vi "Facade.vi"(0 "Data In":T4, 2 "Display State In":T2, 3 "Container State":T3) -> (6 "Data Out":T4, 7 "Display State Out":T2, 8 "Action":T1)   [LabVIEW 2015, in "ToneCloud.xctl"]
uses:
  ToneCloud.xctl
  Data.vi
  Classes/Waveforms/Tone Cloud/Tone Cloud.lvclass
  <vilib>/_xctls/Container State.ctl
  State.vi
  <vilib>/_xctls/Action.ctl
  Classes/Waveforms/Tone Cloud/Tone Cloud.lvclass/Tone Cloud.ctl
  Classes/Waveforms/Tone Cloud/Read Serialized.vi
  Classes/Waveforms/Tone Cloud/Write Serialized.vi
  <vilib>/_xctls/XControlSupport.lvlib
panel:
  in  "Plot mask":bool
  in  "Tokens":i32 min=0
  in  "Seed":i32
  in  "Rate (Hz)":dbl
  in  "Duration (ms)":dbl
  in  "Ramp (ms)":dbl
  in  "Density":string
  in  "Level mode":enum16{"per component", "total rms"}(ring)
  in  "Level (dB)":string
  in  "#/oct":dbl=1.0 min=1.0
  in  "Spacing":enum16{"Linear", "Log"}(ring)
  in  "Fmax (Hz)":dbl
  in  "Fmin (Hz)":dbl
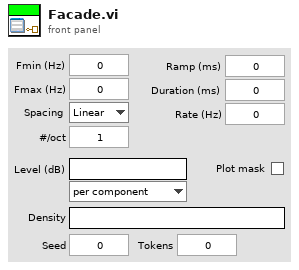
[diagram p1: front panel]
types:
  T1 = typedef "XControlSupport.lvlib/Action.ctl" = cluster{"Data Changed?":bool, "State Changed?":bool, "Action Name":string}
  T2 = typedef "ToneCloud.xctl/State.vi" = cluster{"Numeric":dbl}
  T3 = typedef "XControlSupport.lvlib/Container State.ctl" = cluster{"Indicator?":bool, "Run Mode?":bool, " Refnum":refnum<vi>}
  T4 = typedef "ToneCloud.xctl/Data.vi" = refnum<class "Tone Cloud.lvclass">
  T5 = typedef "Tone Cloud.lvclass/Serialized.ctl" = cluster{"Fmin (Hz)":dbl, "Fmax (Hz)":dbl, "Spacing":T6, "Components/oct":dbl, "Level (dB)":string, "Level mode":T7, "Density":string, "Pip ramp (ms)":dbl, "Pip duration (ms)":dbl, "Pip rate (Hz)":dbl, "Seed":i32, "Tokens":i32, "Plot mask":bool}
  T6 = typedef "Tone Cloud.lvclass/Spacing.ctl" = enum16{"Linear", "Log"}
  T7 = typedef "Tone Cloud.lvclass/Level Mode.ctl" = enum16{"per component", "total rms"}
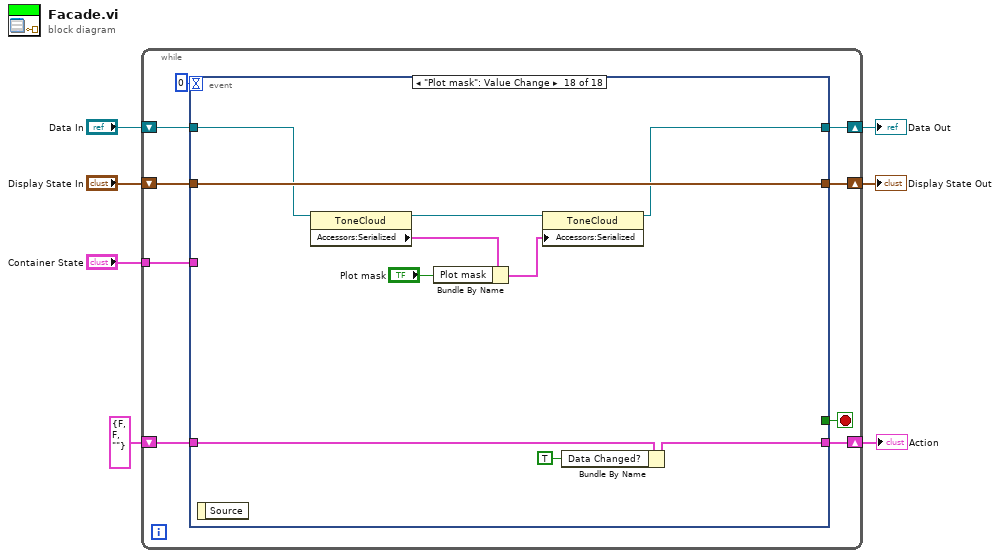
[diagram p0: block diagram]
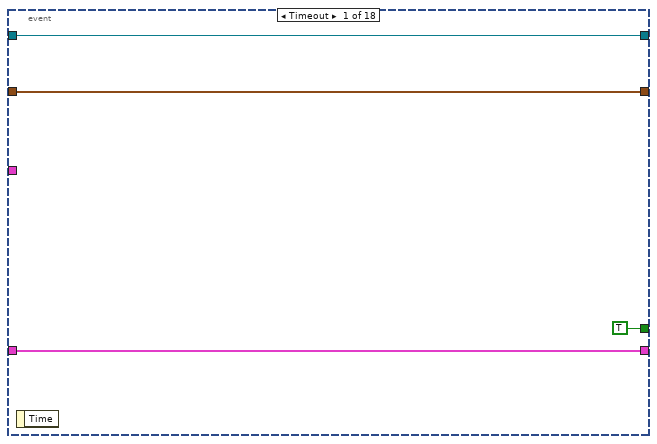
[diagram p2: hidden frame]
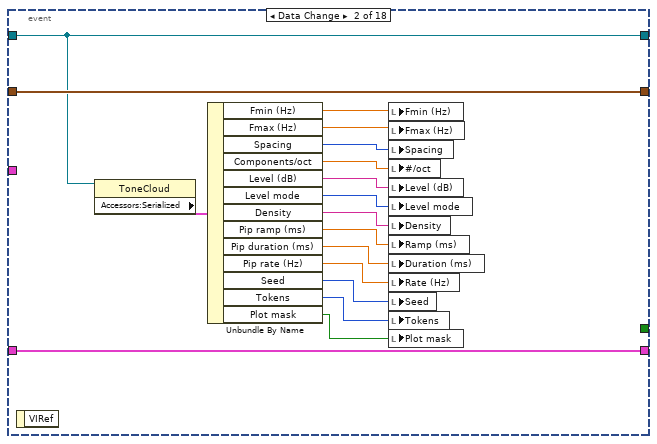
[diagram p3: hidden frame]
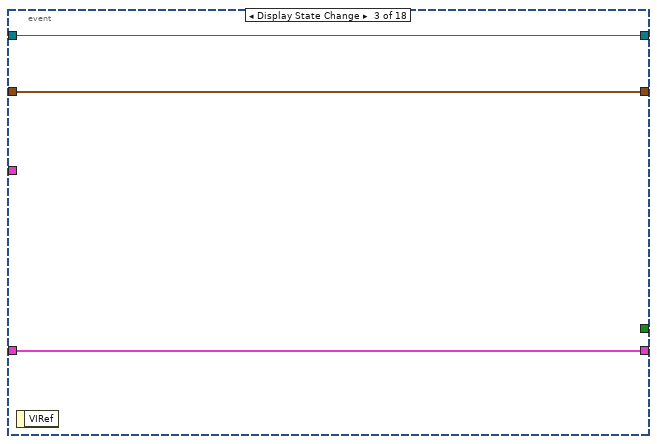
[diagram p4: hidden frame]
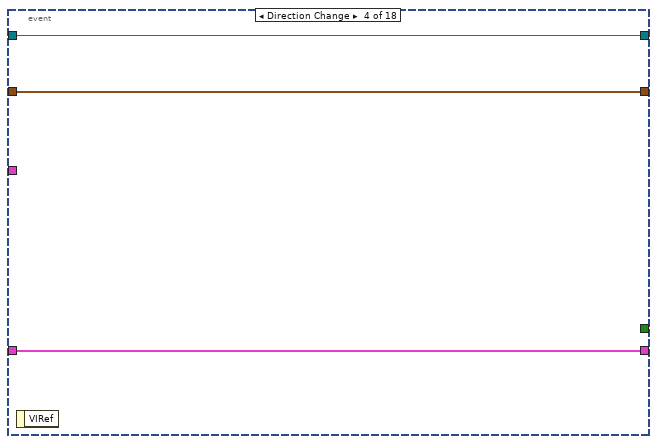
[diagram p5: hidden frame]
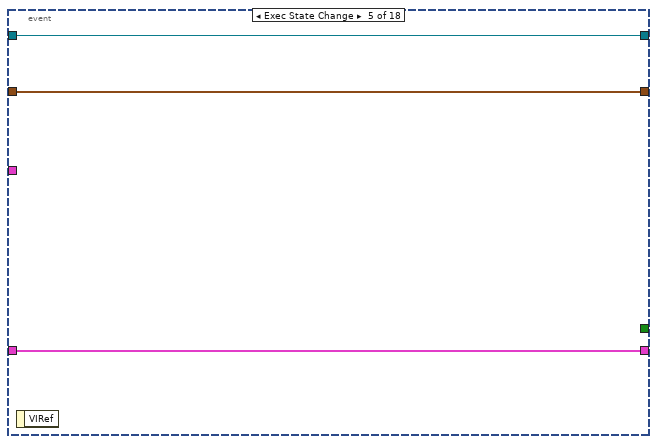
[diagram p6: hidden frame]
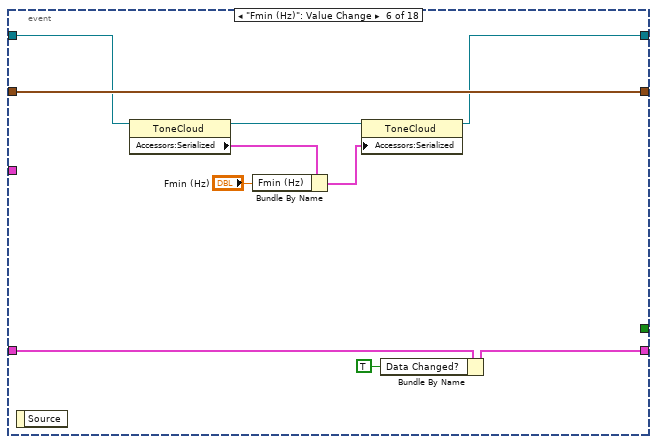
[diagram p7: hidden frame]
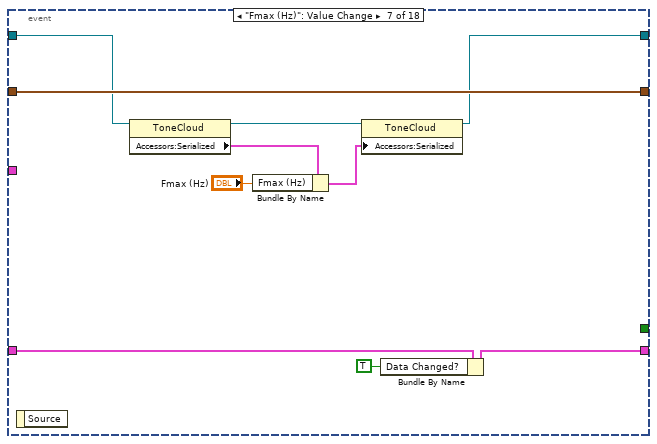
[diagram p8: hidden frame]
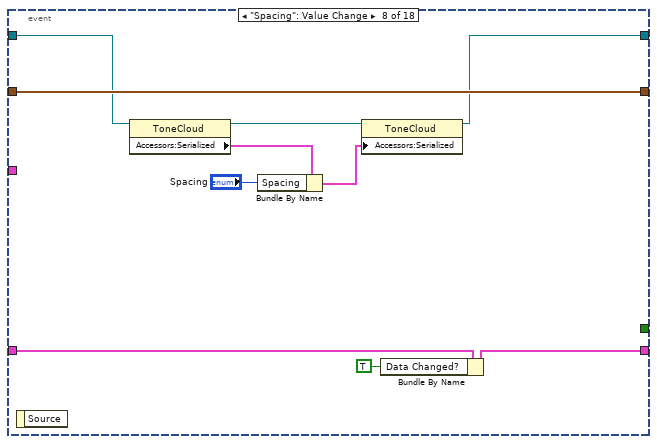
[diagram p9: hidden frame]
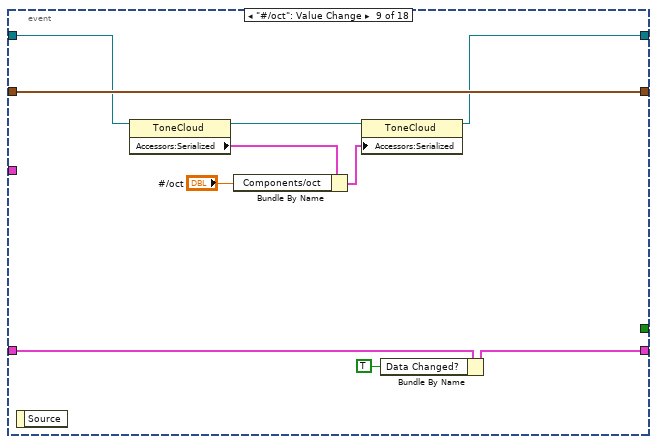
[diagram p10: hidden frame]
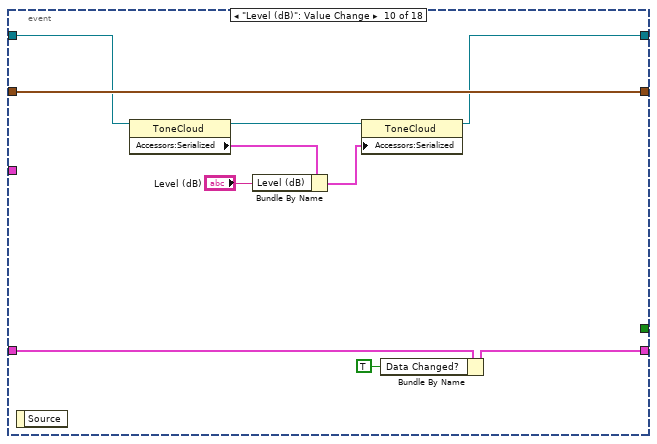
[diagram p11: hidden frame]
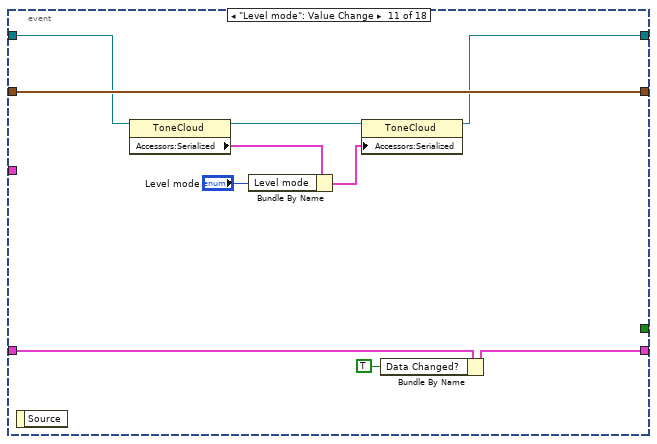
[diagram p12: hidden frame]
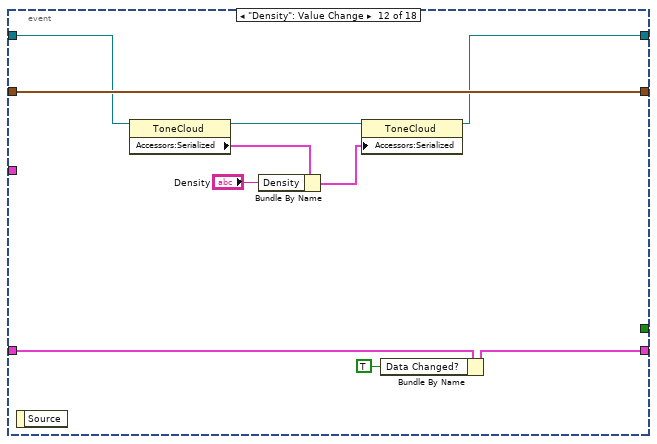
[diagram p13: hidden frame]
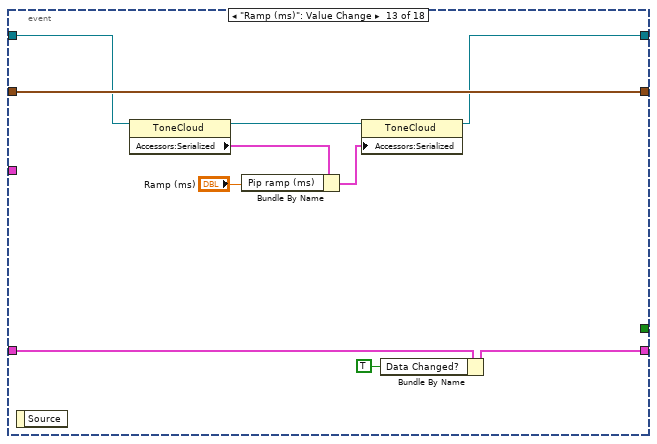
[diagram p14: hidden frame]
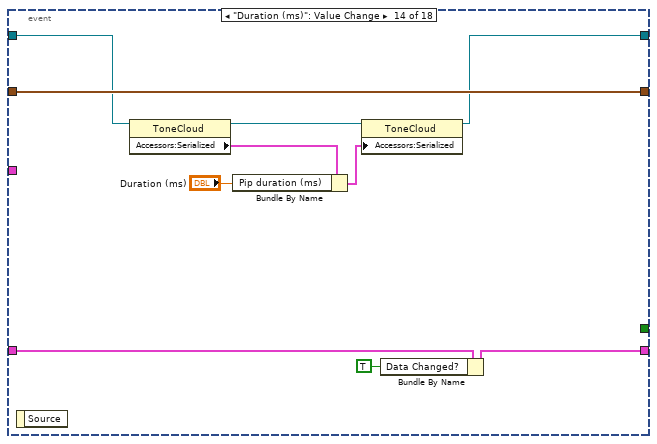
[diagram p15: hidden frame]
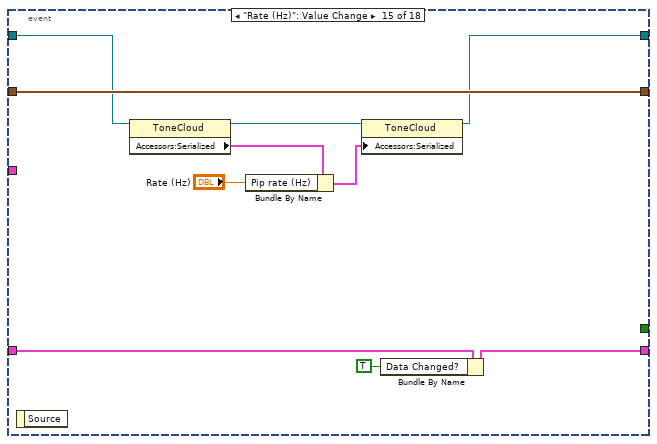
[diagram p16: hidden frame]
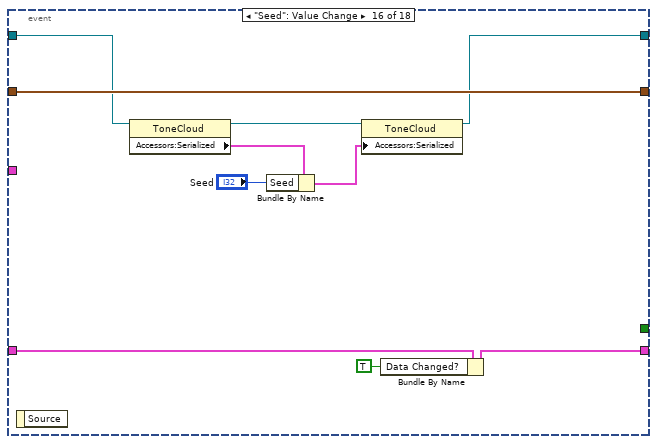
[diagram p17: hidden frame]
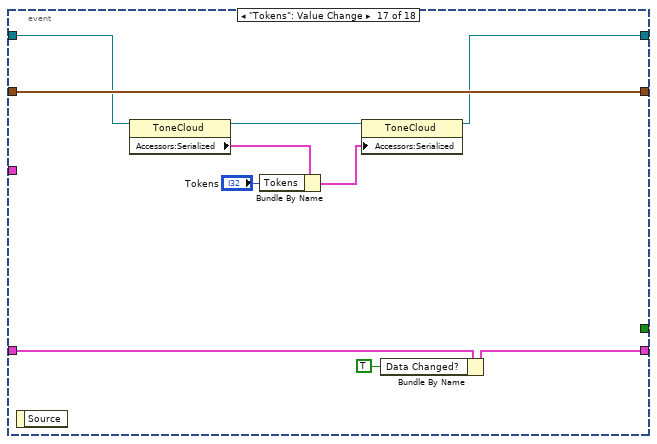
[diagram p18: hidden frame]
diagram:
  n1 = while {
    shift-right: [w15] -> w4
    shift-left: "Display State In" -> [w16]
    tunnel: "Container State" -> [w12]
    shift-right: [w10] -> w7
    shift-left: "Data In" -> [w11]
    shift-right: [w8] -> w2
    shift-left: T1 {"Data Changed?"=FALSE, "State Changed?"=FALSE, "Action Name"=""} ("Action") -> [w9]
    stop <- w14 stop-if-true
    n2 = event shown="[17] \"Plot mask\": Value Change" {
      selector: _ -> [_ _ _ _ _ _ _ _ _ _ _ _ _ _ _ _ _ _]
      dyn-events: _ -> [_ _ _ _ _ _ _ _ _ _ _ _ _ _ _ _ _ _]
      timeout: 0 -> [_ _ _ _ _ _ _ _ _ _ _ _ _ _ _ _ _ _]
      tunnel: w16 -> [w18 w37 w40 w43 w46 w56 w66 w76 w86 w96 w106 w116 w126 w136 w146 w156 w166 w176]
      tunnel: [w18 w37 w40 w43 w46 w56 w66 w76 w86 w96 w106 w116 w126 w136 w146 w156 w166 w176] -> w15
      tunnel: [TRUE _ _ _ _ _ _ _ _ _ _ _ _ _ _ _ _ _] -> w14
      tunnel: w12 -> [_ _ _ _ _ _ _ _ _ _ _ _ _ _ _ _ _ _]
      tunnel: w11 -> [w17 w35 w39 w42 w45 w49 w59 w69 w79 w89 w99 w109 w119 w129 w139 w149 w159 w169]
      tunnel: [w17 w35 w39 w42 w45 w48 w58 w68 w78 w88 w98 w108 w118 w128 w138 w148 w158 w168] -> w10
      tunnel: [w19 w36 w38 w41 w44 w54 w64 w74 w84 w94 w104 w114 w124 w134 w144 w154 w164 w174] -> w8
      tunnel: w9 -> [w19 w36 w38 w41 w44 w55 w65 w75 w85 w95 w105 w115 w125 w135 w145 w155 w165 w175]
      event Timeout {
        n3 = event-data() -> ()  [unwired: 1 in, 1 out]
      }
      event Data Change {
        n4 = event-data() -> ()  [unwired: 1 in, 1 out]
        n5 = property class="ToneCloud"(reference=w35) -> ("Accessors:Serialized"=w34:T5)  [unwired: 1 in, 2 out]
        n6 = Unbundle By Name(w34) -> ("Fmin (Hz)"=w33:dbl, "Fmax (Hz)"=w32:dbl, "Spacing"=w31:T6, "Components/oct"=w30:dbl, "Level (dB)"=w29:string, "Level mode"=w28:T7, "Density"=w27:string, "Pip ramp (ms)"=w26:dbl, "Pip duration (ms)"=w25:dbl, "Pip rate (Hz)"=w24:dbl, "Seed"=w23:i32, "Tokens"=w22:i32, "Plot mask"=w21:bool)
        n7 = local write "Fmin (Hz)"(w33) -> ()
        n8 = local write "Fmax (Hz)"(w32) -> ()
        n9 = local write "Spacing"(w31) -> ()
        n10 = local write "#/oct"(w30) -> ()
        n11 = local write "Level (dB)"(w29) -> ()
        n12 = local write "Level mode"(w28) -> ()
        n13 = local write "Density"(w27) -> ()
        n14 = local write "Ramp (ms)"(w26) -> ()
        n15 = local write "Duration (ms)"(w25) -> ()
        n16 = local write "Rate (Hz)"(w24) -> ()
        n17 = local write "Seed"(w23) -> ()
        n18 = local write "Tokens"(w22) -> ()
        n19 = local write "Plot mask"(w21) -> ()
      }
      event Display State Change {
        n20 = event-data() -> ()  [unwired: 1 in, 1 out]
      }
      event Direction Change {
        n21 = event-data() -> ()  [unwired: 1 in, 1 out]
      }
      event Exec State Change {
        n22 = event-data() -> ()  [unwired: 1 in, 1 out]
      }
      event "Fmin (Hz)": Value Change {
        n23 = event-data() -> ()  [unwired: 1 in, 1 out]
        n24 = property class="ToneCloud"(reference=w49) -> (reference out=w51:T4, "Accessors:Serialized"=w52:T5)  [unwired: 1 in, 1 out]
        n25 = Bundle By Name(cluster=w52, "Fmin (Hz)"="Fmin (Hz)") -> (w50:T5)
        n26 = property class="ToneCloud"(reference=w51, "Accessors:Serialized"=w50) -> (reference out=w48:T4)  [unwired: 1 in, 1 out]
        n27 = Bundle By Name(cluster=w55, "Data Changed?"=TRUE) -> (w54:T1)
      }
      event "Fmax (Hz)": Value Change {
        n28 = event-data() -> ()  [unwired: 1 in, 1 out]
        n29 = property class="ToneCloud"(reference=w59) -> (reference out=w61:T4, "Accessors:Serialized"=w62:T5)  [unwired: 1 in, 1 out]
        n30 = Bundle By Name(cluster=w62, "Fmax (Hz)"="Fmax (Hz)") -> (w60:T5)
        n31 = property class="ToneCloud"(reference=w61, "Accessors:Serialized"=w60) -> (reference out=w58:T4)  [unwired: 1 in, 1 out]
        n32 = Bundle By Name(cluster=w65, "Data Changed?"=TRUE) -> (w64:T1)
      }
      event "Spacing": Value Change {
        n33 = event-data() -> ()  [unwired: 1 in, 1 out]
        n34 = property class="ToneCloud"(reference=w69) -> (reference out=w71:T4, "Accessors:Serialized"=w72:T5)  [unwired: 1 in, 1 out]
        n35 = Bundle By Name(cluster=w72, "Spacing"="Spacing") -> (w70:T5)
        n36 = property class="ToneCloud"(reference=w71, "Accessors:Serialized"=w70) -> (reference out=w68:T4)  [unwired: 1 in, 1 out]
        n37 = Bundle By Name(cluster=w75, "Data Changed?"=TRUE) -> (w74:T1)
      }
      event "#/oct": Value Change {
        n38 = event-data() -> ()  [unwired: 1 in, 1 out]
        n39 = property class="ToneCloud"(reference=w79) -> (reference out=w81:T4, "Accessors:Serialized"=w82:T5)  [unwired: 1 in, 1 out]
        n40 = Bundle By Name(cluster=w82, "Components/oct"="#/oct") -> (w80:T5)
        n41 = property class="ToneCloud"(reference=w81, "Accessors:Serialized"=w80) -> (reference out=w78:T4)  [unwired: 1 in, 1 out]
        n42 = Bundle By Name(cluster=w85, "Data Changed?"=TRUE) -> (w84:T1)
      }
      event "Level (dB)": Value Change {
        n43 = event-data() -> ()  [unwired: 1 in, 1 out]
        n44 = property class="ToneCloud"(reference=w89) -> (reference out=w91:T4, "Accessors:Serialized"=w92:T5)  [unwired: 1 in, 1 out]
        n45 = Bundle By Name(cluster=w92, "Level (dB)"="Level (dB)") -> (w90:T5)
        n46 = property class="ToneCloud"(reference=w91, "Accessors:Serialized"=w90) -> (reference out=w88:T4)  [unwired: 1 in, 1 out]
        n47 = Bundle By Name(cluster=w95, "Data Changed?"=TRUE) -> (w94:T1)
      }
      event "Level mode": Value Change {
        n48 = event-data() -> ()  [unwired: 1 in, 1 out]
        n49 = property class="ToneCloud"(reference=w99) -> (reference out=w101:T4, "Accessors:Serialized"=w102:T5)  [unwired: 1 in, 1 out]
        n50 = Bundle By Name(cluster=w102, "Level mode"="Level mode") -> (w100:T5)
        n51 = property class="ToneCloud"(reference=w101, "Accessors:Serialized"=w100) -> (reference out=w98:T4)  [unwired: 1 in, 1 out]
        n52 = Bundle By Name(cluster=w105, "Data Changed?"=TRUE) -> (w104:T1)
      }
      event "Density": Value Change {
        n53 = event-data() -> ()  [unwired: 1 in, 1 out]
        n54 = property class="ToneCloud"(reference=w109) -> (reference out=w111:T4, "Accessors:Serialized"=w112:T5)  [unwired: 1 in, 1 out]
        n55 = Bundle By Name(cluster=w112, "Density"="Density") -> (w110:T5)
        n56 = property class="ToneCloud"(reference=w111, "Accessors:Serialized"=w110) -> (reference out=w108:T4)  [unwired: 1 in, 1 out]
        n57 = Bundle By Name(cluster=w115, "Data Changed?"=TRUE) -> (w114:T1)
      }
      event "Ramp (ms)": Value Change {
        n58 = event-data() -> ()  [unwired: 1 in, 1 out]
        n59 = property class="ToneCloud"(reference=w119) -> (reference out=w121:T4, "Accessors:Serialized"=w122:T5)  [unwired: 1 in, 1 out]
        n60 = Bundle By Name(cluster=w122, "Pip ramp (ms)"="Ramp (ms)") -> (w120:T5)
        n61 = property class="ToneCloud"(reference=w121, "Accessors:Serialized"=w120) -> (reference out=w118:T4)  [unwired: 1 in, 1 out]
        n62 = Bundle By Name(cluster=w125, "Data Changed?"=TRUE) -> (w124:T1)
      }
      event "Duration (ms)": Value Change {
        n63 = event-data() -> ()  [unwired: 1 in, 1 out]
        n64 = property class="ToneCloud"(reference=w129) -> (reference out=w131:T4, "Accessors:Serialized"=w132:T5)  [unwired: 1 in, 1 out]
        n65 = Bundle By Name(cluster=w132, "Pip duration (ms)"="Duration (ms)") -> (w130:T5)
        n66 = property class="ToneCloud"(reference=w131, "Accessors:Serialized"=w130) -> (reference out=w128:T4)  [unwired: 1 in, 1 out]
        n67 = Bundle By Name(cluster=w135, "Data Changed?"=TRUE) -> (w134:T1)
      }
      event "Rate (Hz)": Value Change {
        n68 = event-data() -> ()  [unwired: 1 in, 1 out]
        n69 = property class="ToneCloud"(reference=w139) -> (reference out=w141:T4, "Accessors:Serialized"=w142:T5)  [unwired: 1 in, 1 out]
        n70 = Bundle By Name(cluster=w142, "Pip rate (Hz)"="Rate (Hz)") -> (w140:T5)
        n71 = property class="ToneCloud"(reference=w141, "Accessors:Serialized"=w140) -> (reference out=w138:T4)  [unwired: 1 in, 1 out]
        n72 = Bundle By Name(cluster=w145, "Data Changed?"=TRUE) -> (w144:T1)
      }
      event "Seed": Value Change {
        n73 = event-data() -> ()  [unwired: 1 in, 1 out]
        n74 = property class="ToneCloud"(reference=w149) -> (reference out=w151:T4, "Accessors:Serialized"=w152:T5)  [unwired: 1 in, 1 out]
        n75 = Bundle By Name(cluster=w152, "Seed"="Seed") -> (w150:T5)
        n76 = property class="ToneCloud"(reference=w151, "Accessors:Serialized"=w150) -> (reference out=w148:T4)  [unwired: 1 in, 1 out]
        n77 = Bundle By Name(cluster=w155, "Data Changed?"=TRUE) -> (w154:T1)
      }
      event "Tokens": Value Change {
        n78 = event-data() -> ()  [unwired: 1 in, 1 out]
        n79 = property class="ToneCloud"(reference=w159) -> (reference out=w161:T4, "Accessors:Serialized"=w162:T5)  [unwired: 1 in, 1 out]
        n80 = Bundle By Name(cluster=w162, "Tokens"="Tokens") -> (w160:T5)
        n81 = property class="ToneCloud"(reference=w161, "Accessors:Serialized"=w160) -> (reference out=w158:T4)  [unwired: 1 in, 1 out]
        n82 = Bundle By Name(cluster=w165, "Data Changed?"=TRUE) -> (w164:T1)
      }
      event "Plot mask": Value Change {
        n83 = event-data() -> ()  [unwired: 1 in, 1 out]
        n84 = property class="ToneCloud"(reference=w169) -> (reference out=w171:T4, "Accessors:Serialized"=w172:T5)  [unwired: 1 in, 1 out]
        n85 = Bundle By Name(cluster=w172, "Plot mask"="Plot mask") -> (w170:T5)
        n86 = property class="ToneCloud"(reference=w171, "Accessors:Serialized"=w170) -> (reference out=w168:T4)  [unwired: 1 in, 1 out]
        n87 = Bundle By Name(cluster=w175, "Data Changed?"=TRUE) -> (w174:T1)
      }
    }
  }
  "Display State Out" <- w4
  "Data Out" <- w7
  "Action" <- w2
